vi "WriteSymbol.vi"(8 "error in (no error)":errorcluster, 9 "tbValue":string caption="Value:", 10 "SymbolName":string, 11 "TCatAdsNet.lvlib:AdsNET.lvclass":refnum<class "AdsNET.lvclass">) -> (0 "error out":errorcluster, 3 "TCatAdsNet.lvlib:AdsNET.lvclass 2":refnum<class "AdsNET.lvclass">)   [LabVIEW 2016, in "TCatAdsNet.lvlib" / "AdsNET.lvclass"]
uses:
  AdsNET.lvclass
  AdsNET.lvclass/AdsNET.ctl
  C:/Users/Maurizio/Projects/twincat-lv-ads-library/TCatAdsNet Library/TwinCAT.Ads.dll
  TwinCAT.Ads.dll
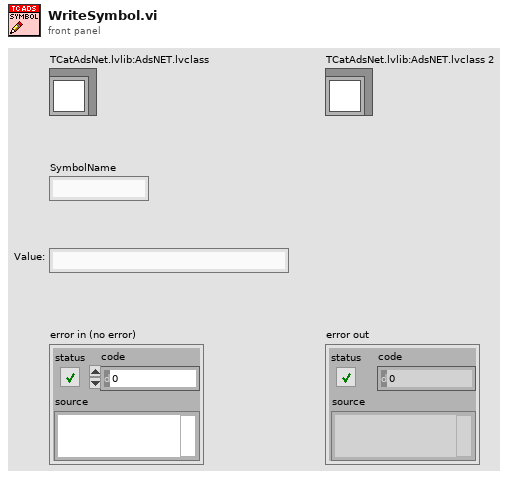
[diagram p1: front panel]
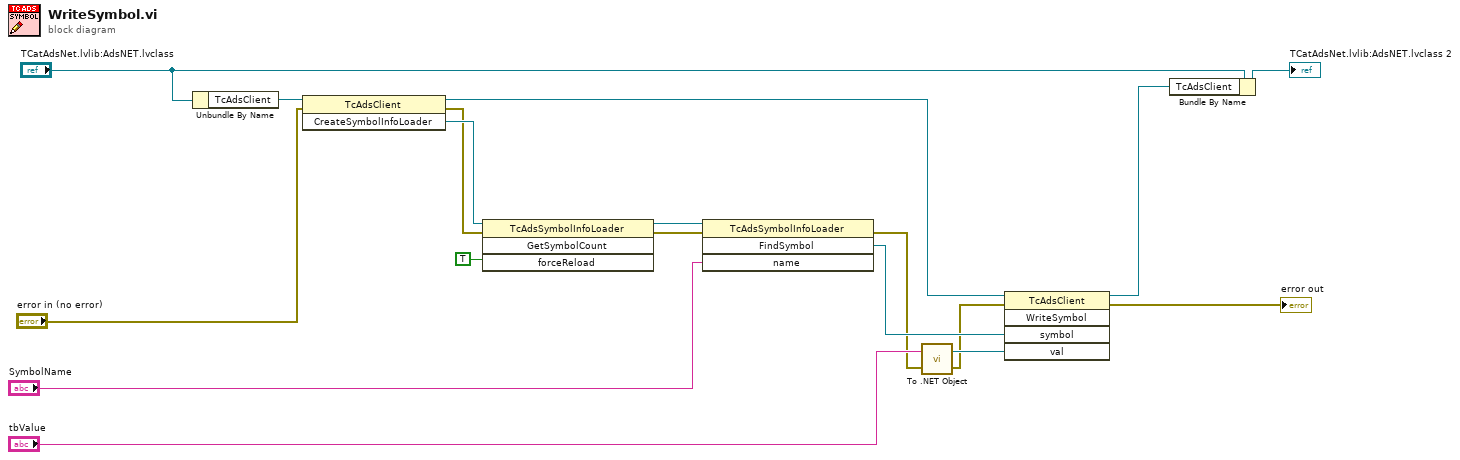
[diagram p0: block diagram]
diagram:
  n1 = Unbundle By Name("TCatAdsNet.lvlib:AdsNET.lvclass") -> ("TcAdsClient"=w6:refnum<k24>)
  n2 = invoke class="TcAdsClient" method="CreateSymbolInfoLoader"(reference=w6, error in="error in (no error)") -> (reference out=w5:refnum<k24>, error out=w7:errorcluster, "CreateSymbolInfoLoader"=w8:refnum<k24>)  [unwired: 1 in]
  n3 = invoke class="TcAdsSymbolInfoLoader" method="GetSymbolCount"(reference=w8, error in=w7, "forceReload"=TRUE) -> (reference out=w2:refnum<k24>, error out=w1:errorcluster)  [unwired: 1 in, 2 out]
  n4 = invoke class="TcAdsSymbolInfoLoader" method="FindSymbol"(reference=w2, error in=w1, "name"="SymbolName") -> (error out=w12:errorcluster, "FindSymbol"=w13:refnum<k24>)  [unwired: 1 in, 2 out]
  n5 = call <vilib>:"To .NET Object.vi"("error in (no error)"=w12, "anything"="tbValue") -> ("error out"=w11:errorcluster, ".NET object"=w18:refnum<k24>)
  n6 = invoke class="TcAdsClient" method="WriteSymbol"(reference=w5, error in=w11, "symbol"=w13, "val"=w18) -> (reference out=w15:refnum<k24>, error out=→"error out":errorcluster)  [unwired: 1 in, 3 out]
  n7 = Bundle By Name(cluster="TCatAdsNet.lvlib:AdsNET.lvclass", "TcAdsClient"=w15) -> (→"TCatAdsNet.lvlib:AdsNET.lvclass 2":refnum<class "AdsNET.lvclass">)
